vi "Close_Reference.vi"(8 "error in":errorcluster, 9 "enable VI checksums":bool, 10 "remove VI object":u16, 11 "AB_Source in":refnum<class "AB_Source.lvclass">) -> (0 "error out":errorcluster, 1 "saveLevel":u32, 2 "checksum":string, 3 "AB_Source out":refnum<class "AB_Source.lvclass">, 4 "Library":refnum<vi>, 6 "VI":refnum<vi>)   [LabVIEW 2020, in "AB_Source.lvclass"]
uses:
  <vilib>/AppBuilder/AB_Classes/Source/AB_Source.lvclass
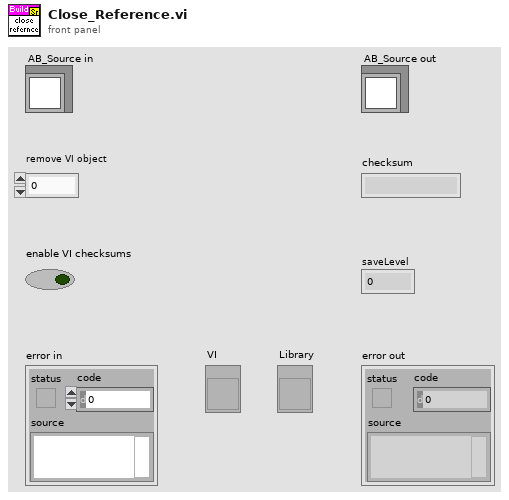
[diagram p1: front panel]
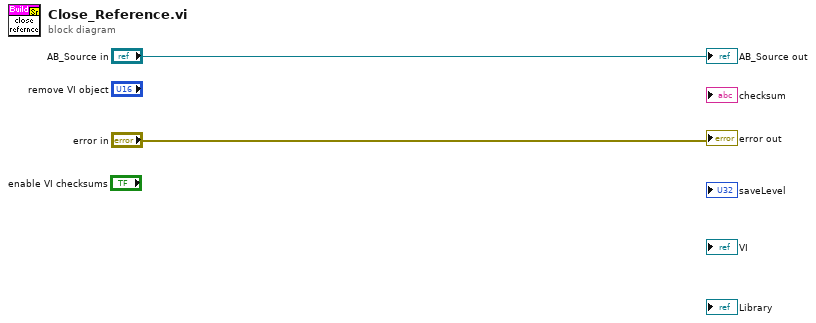
[diagram p0: block diagram]
diagram:
  "error out" <- "error in"
  "AB_Source out" <- "AB_Source in"
